vi "Add Subaddress.vi"(8 "error in":errorcluster, 9 "direction":T1, 10 "subaddress":T2, 11 "remote terminal":T3 format="%.0x") -> (0 "error out":errorcluster, 2 "subaddress section":T3 format="%.0x", 3 "remote terminal out":T3 format="%.0x")   [LabVIEW 2020, in "AIM MIL-STD-1553 Scripting.lvlib"]
doc: "Adds a <b>subaddress section</b> to the <b>remote terminal</b> and sets it to contain the specified <b>subaddress</b> value."
uses:
  AIM MIL-STD-1553 Scripting.lvlib
  <vilib>/NI VeriStand/Custom Device API/Custom Device Item Ref.ctl
  Shared/Address.ctl
  Shared/Direction.ctl
  Constants.vi
  GlobalVariables.vi
  <vilib>/NI VeriStand/Custom Device API/Custom Device API.lvlib
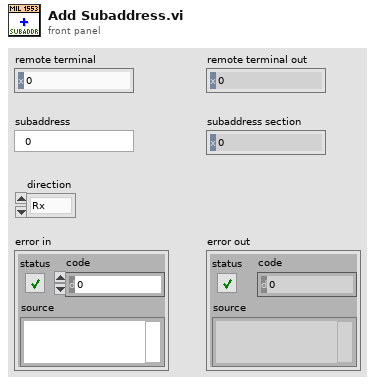
[diagram p1: front panel]
types:
  T1 = typedef "Direction.ctl" = enum16{"Rx", "Tx"}
  T2 = typedef "Address.ctl" = u16
  T3 = typedef "Custom Device API.lvlib/Custom Device Item Ref.ctl" = u64
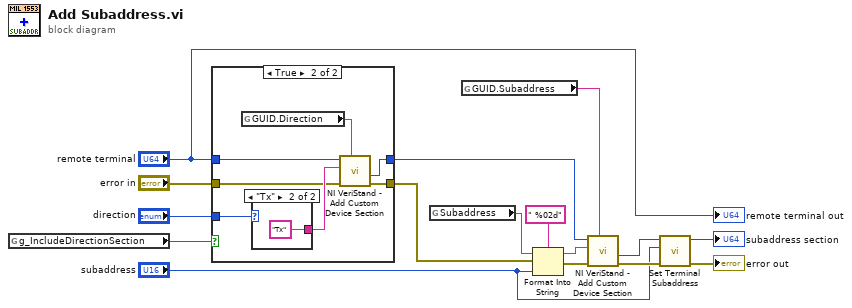
[diagram p0: block diagram]
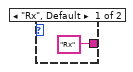
[diagram p3: hidden frame]
diagram:
  n1 = global read "GlobalVariables.vi" "g_IncludeDirectionSection"() -> (w1:bool)
  n2 = case shown="True" w1 {
    tunnel: "direction" -> [_ w25]
    tunnel: "error in" -> [w18 w23]
    tunnel: [w18 w22] -> w5
    tunnel: "remote terminal" -> [w17 w21]
    tunnel: [w17 w20] -> w4
    frame False {
    }
    frame True {
      n3 = global read "Constants.vi" "GUID.Direction"() -> (w19:string)
      n4 = case shown="\"Tx\"" w25 {
        tunnel: ["Rx" "Tx"] -> w24
        frame "Rx", Default {
        }
        frame "Tx" {
        }
      }
      n5 = call <vilib>:"NI VeriStand - Add Custom Device Section.vi"("GUID (Default Section)"=w19, "error in (no error)"=w23, "Section Name"=w24, "Parent Ref in"=w21) -> ("error out"=w22:errorcluster, "Section Ptr"=w20:T3)  [unwired: 4 in, 2 out]
    }
  }
  n6 = global read "Constants.vi" "Subaddress"() -> (w10:string)
  n7 = global read "Constants.vi" "GUID.Subaddress"() -> (w16:string)
  n8 = Format Into String(format string=" %02d", initial string=w10, error in=w5, "subaddress") -> (resulting string=w12:string, error out=w11:errorcluster)
  n9 = call <vilib>:"NI VeriStand - Add Custom Device Section.vi"("GUID (Default Section)"=w16, "error in (no error)"=w11, "Section Name"=w12, "Parent Ref in"=w4) -> ("error out"=w14:errorcluster, "Section Ptr"=w9:T3)  [unwired: 4 in, 2 out]
  n10 = call "Set Terminal Subaddress.vi"("error in"=w14, "subaddress"="subaddress", "subaddress section"=w9) -> ("error out"=→"error out":errorcluster, "subaddress section out"=→"subaddress section":T3)  [unwired: 7 in]
  "remote terminal out" <- "remote terminal"
